vi "AVS_Set_excitation.vi"() -> ()   [LabVIEW 2018]
uses:
  Instrument_Setup.vi
panel:
  out "error out (no error) 2":errorcluster
  in  "error in (no error) 3":errorcluster
  in  "Delay (sec) 2":i16=1 min=0 max=3600 step=1
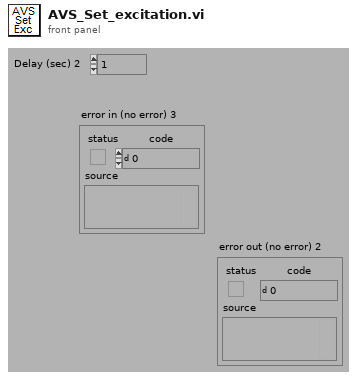
[diagram p1: front panel]
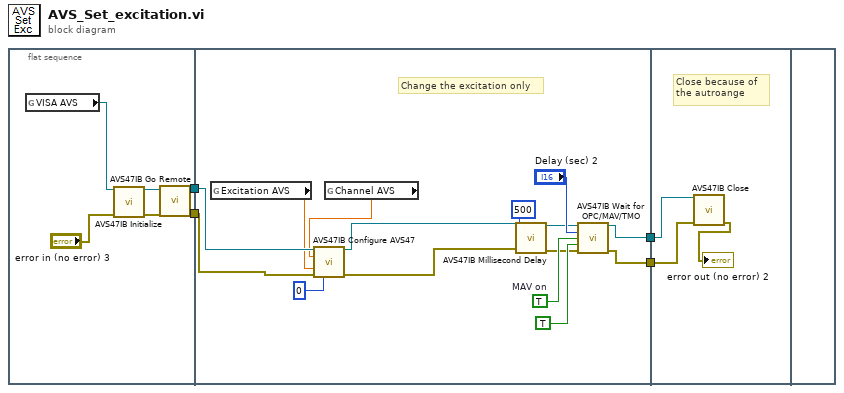
[diagram p0: block diagram]
diagram:
  n1 = flat-sequence {
    tunnel: [w7] -> w4
    tunnel: [w6] -> w3
    tunnel: [w16] -> w2
    tunnel: [w15] -> w1
    tunnel: w4 -> [w14]
    tunnel: w3 -> [w13]
    tunnel: w2 -> [w27]
    tunnel: w1 -> [w26]
    frame #0 {
      n2 = global read "Instrument_Setup.vi" "VISA AVS"() -> (w5:refnum<visa-resource-name>)
      n3 = call "AVS47IB Initialize.vi"("VISA session (for class)"=w5, "error in (no error)"="error in (no error) 3") -> ("VISA session"=w9:refnum<visa-resource-name>, "error out"=w8:errorcluster)  [unwired: 12 in]
      n4 = call "AVS47IB Go Remote.vi"("VISA session"=w9, "error in (no error)"=w8) -> ("dup VISA session"=w7:refnum<visa-resource-name>, "error out"=w6:errorcluster)  [unwired: 12 in]
    }
    frame #1 {
      w24 = TRUE  # MAV on
      # "Change the excitation only"
      n5 = global read "Instrument_Setup.vi" "Excitation AVS"() -> (w12:dbl)
      n6 = global read "Instrument_Setup.vi" "Channel AVS"() -> (w11:dbl)
      n7 = call "AVS47IB Configure AVS47.vi"("VISA session"=w14, "CHANNEL (-1:no change )"=w11, "EXCITATION (-1:no change)"=w12, "error in (no error)"=w13, "DISPLAY (-1:no change)"=i8 0) -> ("dup VISA session"=w18:refnum<visa-resource-name>, "error out"=w17:errorcluster)  [unwired: 9 in]
      n8 = call "AVS47IB Millisecond Delay.vi"("VISA session"=w18, "Delay (50 ms)"=500, "error in (no error)"=w17) -> ("dup VISA session"=w21:refnum<visa-resource-name>, "error out"=w20:errorcluster)  [unwired: 11 in]
      n9 = call "AVS47IB Wait for OPC/MAV/TMO.vi"("VISA session"=w21, "Timeout (2 sec)"="Delay (sec) 2", "MAV (on)"=w24, "OPC (off)"=TRUE, "error in (no error)"=w20) -> ("dup VISA session"=w16:refnum<visa-resource-name>, "error out"=w15:errorcluster)  [unwired: 8 in, 1 out]
    }
    frame #2 {
      # "Close because of \nthe autroange"
      n10 = call "AVS47IB Close.vi"("VISA session"=w27, "error in (no error)"=w26) -> ("error out"=→"error out (no error) 2":errorcluster)  [unwired: 13 in]
    }
    frame #3 {
    }
  }
